vi "VIQA Time Elapsed.vi"(7 "Auto Reset (T)":bool=TRUE, 10 "Reset (F)":bool, 11 "Duration (1 sec)":dbl=1.0) -> (2 "Elapsed Time (sec)":dbl, 3 "Time Has Elapsed?":bool)   [LabVIEW 2018, in "VI Quality.lvlib"]
doc: "This VI calculates and indicates the time elapsed given the duration in seconds. Set Auto Reset to restart the timer."
uses:
  VI Quality.lvlib
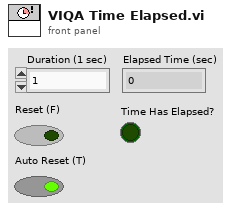
[diagram p1: front panel]
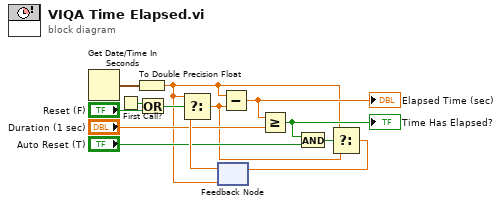
[diagram p0: block diagram]
diagram:
  n1 = Get Date/Time In Seconds() -> (seconds since 1Jan1904=w3:timestamp)
  n2 = First Call?() -> (First Call?: T/F=w11:bool)
  n3 = To Double Precision Float(number=w3) -> (double precision float=w1:dbl)
  n4 = Or(x=w11, y="Reset (F)") -> (x .or. y?=w2:bool)
  n5 = feedback #1(w1) -> (w12:dbl)
  n6 = Select(t=w1, s=w2, f=w12) -> (s? t:f=w5:dbl)
  n7 = Subtract(x=w1, y=w5) -> (x-y=w6:dbl)
  "Elapsed Time (sec)" <- w6
  n8 = Greater Or Equal?(x=w6, y="Duration (1 sec)") -> (x >= y?=w8:bool)
  "Time Has Elapsed?" <- w8
  n9 = And(x=w8, y="Auto Reset (T)") -> (x .and. y?=w4:bool)
  n10 = Select(t=w1, s=w4, f=w5) -> (s? t:f=w13:dbl)
  n11 = feedback-in #1(w13) -> ()
